vi "get 3x3.vi"(1 "input":i32[][](array[numeric]), 2 "COL 2":i32, 3 "COL 1":i32, 4 "ROW 2":i32, 5 "ROW 1":i32) -> (0 "output":i32[][](array[numeric]))   [LabVIEW 2014]
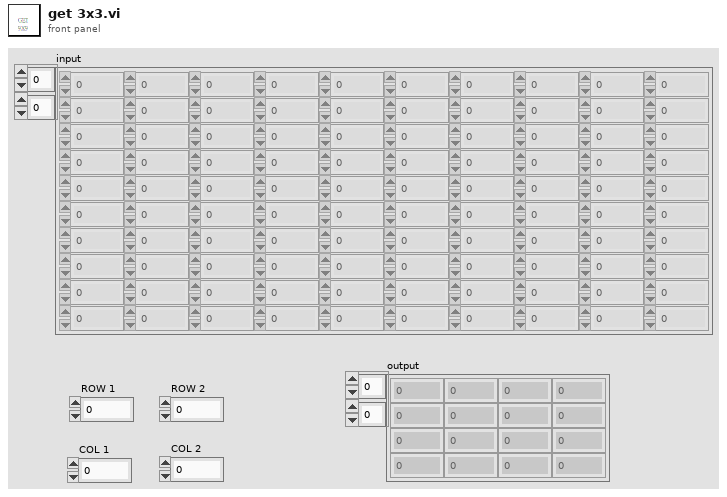
[diagram p1: front panel]
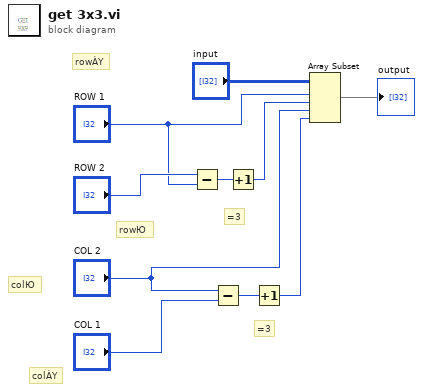
[diagram p0: block diagram]
diagram:
  # "=3"
  # "=3"
  # "colÀY"
  # "colЮ"
  # "rowЮ"
  # "rowÀY"
  n1 = Subtract(x="ROW 2", y="ROW 1") -> (x-y=w10:i32)
  n2 = Subtract(x="COL 2", y="COL 1") -> (x-y=w8:i32)
  n3 = Increment(x=w10) -> (x+1=w9:i32)
  n4 = Increment(x=w8) -> (x+1=w7:i32)
  n5 = Array Subset(array="input", index (row)="ROW 1", length (row)=w9, index (col)="COL 2", length (col)=w7) -> (→"output":i32[][])
